vi "Receive and Broadcast Event.vi"(8 "error in (no error)":errorcluster, 9 "Event Data":refnum<class "Event.lvclass">, 10 "Sink Enqueuer":refnum<class "Message Enqueuer.lvclass">, 11 "Event Source in":refnum<class "Event Source.lvclass">) -> (0 "error out":errorcluster, 3 "Event Source out":refnum<class "Event Source.lvclass">)   [LabVIEW 2016, in "Event Source.lvlib" / "Event Source.lvclass"]
doc: "This method generates/fires the Event wired to the input triggered by a Sink Actor. Firing an event originating form a Sink Actor looks up all actors, but the originating Sink, who Registered to listen to this Event and sends to them this Event on a Zero Coupling based message defined during Registration. Errors on broadcasting the event i.e. enqueuer of the registrant not existing, are ignored.\n\n<b>IMPORTANT</b> - Only call this method within actor core of your Event Source Actor. From helper loops call the Send Generate Event message to self. This is to make sure your actor works with all registered listeners.a"
uses:
  Event Source.lvclass
  <vilib>/ActorFramework/Message Enqueuer/Message Enqueuer.lvclass
  Event/Event.lvclass
  Event Source.lvclass/Event Source.ctl
  Event Handler Details.ctl
  Event Source Messages/Event Generated Msg/Event Generated Msg.lvclass
  C:/Program Files (x86)/National Instruments/LabVIEW 2016/vi.lib/ActorFramework/Message/Message.lvclass
  Event Source Messages/Event Generated Msg/Event Generated Msg.lvclass/Event Generated Msg.ctl
  <vilib>/ActorFramework/Message Enqueuer/Message Enqueuer.lvclass/Message Enqueuer.ctl
  <vilib>/ActorFramework/Message Enqueuer/Enqueue.vi
  <vilib>/Utility/LVClass/Get LV Class Name.vi
  <resource>/AFDebug/Generate Trace for Message.vi
  <vilib>/ActorFramework/Message Priority Queue/Priority Enqueue.vi
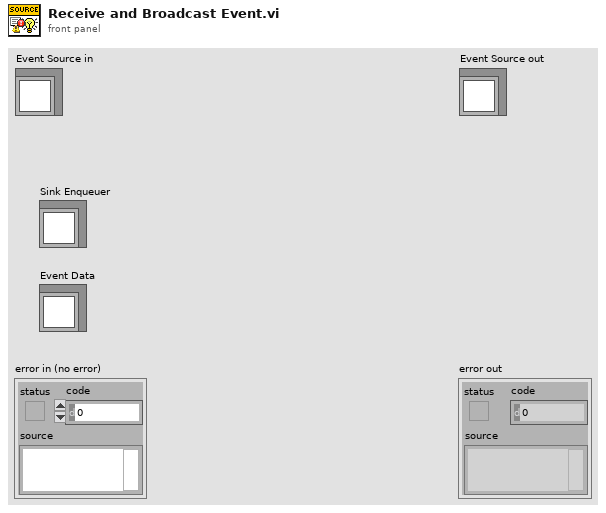
[diagram p1: front panel]
types:
  T1 = typedef "Event Source.lvlib/Event Source.lvclass/Event Handler Details.ctl" = cluster{"Exclude From Broadcast":bool, "Paused":bool, "Sink Event Fire Handler":refnum<class "Event Generated Msg.lvclass">}
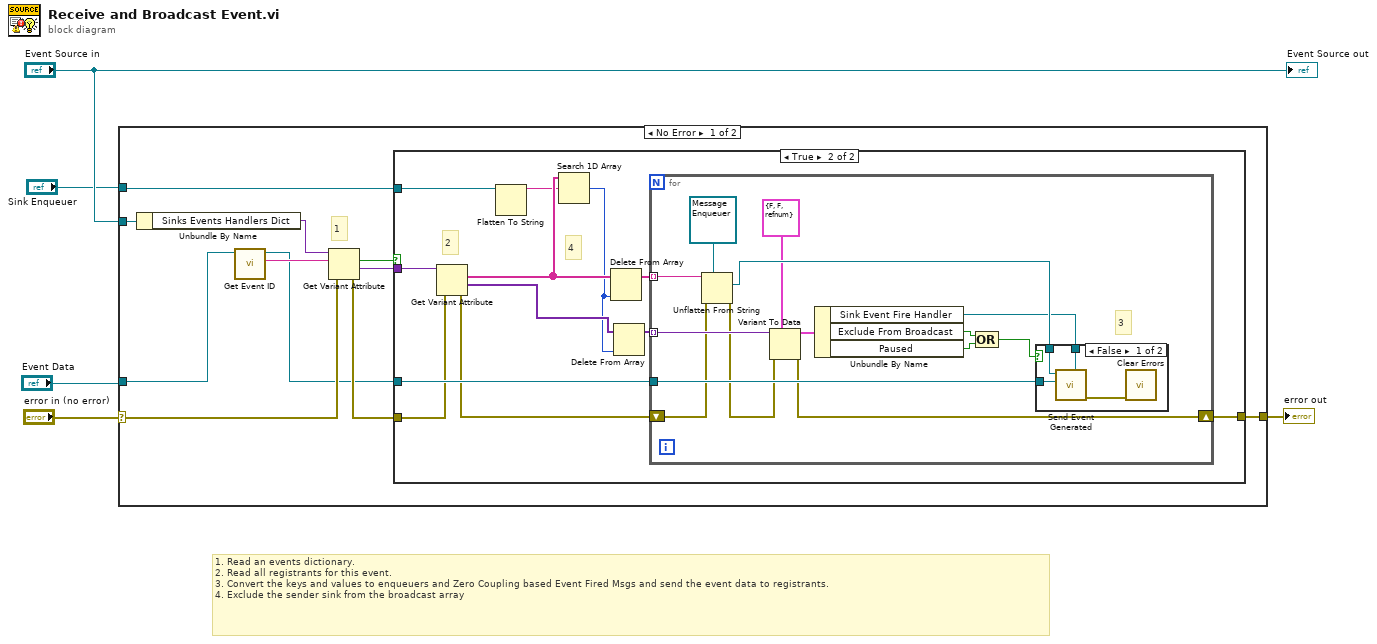
[diagram p0: block diagram]
diagram:
  # "1. Read an events dictionary.\n2. Read all registrants for this event.\n3. Convert the keys and values to enqueuers and Zero Coupling based Event Fired Msgs and send the event data to registrants.\n4. Exclude the sender sink from the broadcast array"
  n1 = case shown="No Error" "error in (no error)" {
    selector: "error in (no error)" -> [w8 w48]
    tunnel: "Event Source in" -> [w16 _]
    tunnel: "Event Data" -> [w10 _]
    tunnel: [w15 w48] -> w1
    tunnel: "Sink Enqueuer" -> [w6 _]
    frame No Error {
      # "1"
      n2 = Unbundle By Name(w16) -> ("Sinks Events Handlers Dict"=w14:variant)
      n3 = call-dynamic "Get Event ID.vi"("Event in"=w10) -> ("Event ID"=w9:string, "Event out"=w7:refnum<class "Event.lvclass">)  [unwired: 8 in, 1 out]
      n4 = Get Variant Attribute(Variant=w14, name=w9, error in=w8) -> (found=w11:bool, value=w12:variant, error out=w13:errorcluster)  [unwired: 1 in, 1 out]
      n5 = case shown="True" w11 {
        tunnel: w12 -> [_ w27]
        tunnel: w7 -> [_ w29]
        tunnel: w13 -> [w17 w26]
        tunnel: [w17 w28] -> w15
        tunnel: w6 -> [_ w22]
        frame False {
        }
        frame True {
          # "4"
          # "2"
          n6 = Get Variant Attribute(Variant=w27, error in=w26) -> (names=w24:string[], values=w20:variant[], error out=w25:errorcluster)  [unwired: 2 in, 1 out]
          n7 = Flatten To String(anything=w22) -> (data string=w21:string)  [unwired: 3 in, 2 out]
          n8 = Search 1D Array(1D array=w24, element=w21) -> (index of element=w18:i32)  [unwired: 1 in]
          n9 = Delete From Array(array=w24, index=w18) -> (array with subset deleted=w23:string[])  [unwired: 1 in, 1 out]
          n10 = Delete From Array(array=w20, index=w18) -> (array with subset deleted=w19:variant[])  [unwired: 1 in, 1 out]
          n11 = for {
            tunnel: w23 -> [w43] mode=indexing
            tunnel: w19 -> [w42] mode=indexing
            tunnel: w29 -> [w39]
            shift-right: [w34] -> w28
            shift-left: w25 -> [w38]
            # "3"
            n12 = Unflatten From String(type=refnum<class "Message Enqueuer.lvclass"> refnum ("Message Enqueuer"), binary string=w43, error in (no error)=w38) -> (value=w41:refnum<class "Message Enqueuer.lvclass">, error out=w37:errorcluster)  [unwired: 2 in, 1 out]
            n13 = Variant To Data(error in=w37, type=T1 {"Exclude From Broadcast"=FALSE, "Paused"=FALSE, "Sink Event Fire Handler"=refnum} ("Message Type"), Variant=w42) -> (data=w40:T1, error out=w34:errorcluster)
            n14 = Unbundle By Name(w40) -> ("Sink Event Fire Handler"=w32:refnum<class "Event Generated Msg.lvclass">, "Exclude From Broadcast"=w31:bool, "Paused"=w30:bool)
            n15 = Compound Arithmetic op=OR(w31, w30) -> (w33:bool)
            n16 = case shown="False" w33 {
              tunnel: w32 -> [w47 _]
              tunnel: w39 -> [w46 _]
              tunnel: w41 -> [w44 _]
              frame False {
                n17 = call "Send Event Generated.vi"("Message Type"=w47, "Event Data"=w46, "Message Enqueuer"=w44) -> ("Error Out"=w45:errorcluster)  [unwired: 7 in, 1 out]
                n18 = call <vilib>:"Clear Errors.vi"("error in (no error)"=w45) -> ()  [unwired: 5 in, 2 out]
              }
              frame True {
              }
            }
          }
        }
      }
    }
    frame Error {
    }
  }
  "error out" <- w1
  "Event Source out" <- "Event Source in"
